vi "Gera_Dmd_Frame.vi"(8 "i":i32, 9 "c_Stop":bool, 11 "A2K - RT":dbl[](array[numeric])) -> (3 "a2c_serial":u8[](array[numeric]))   [LabVIEW 2011]
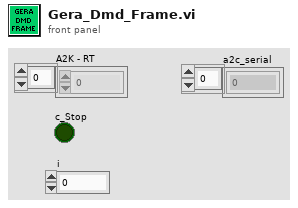
[diagram p1: front panel]
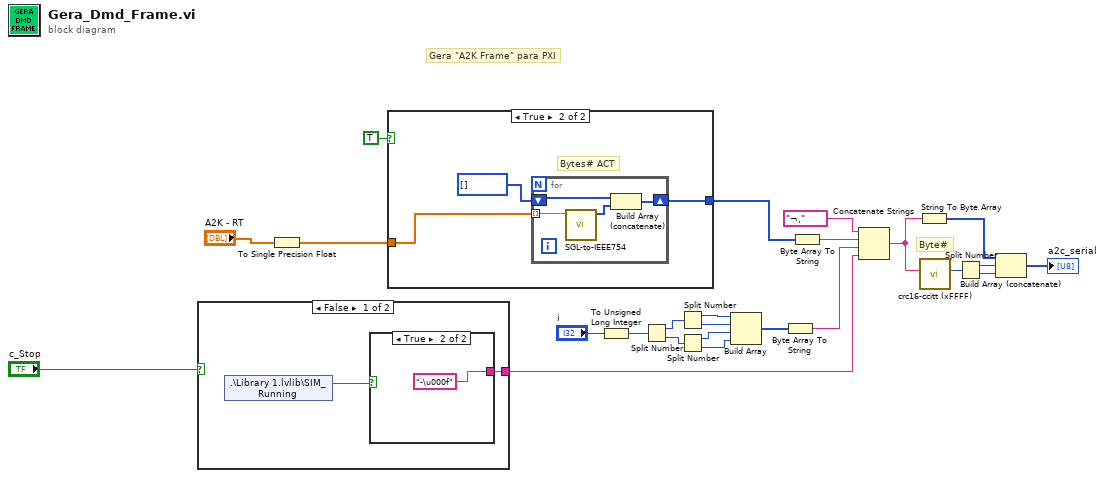
[diagram p0: block diagram]
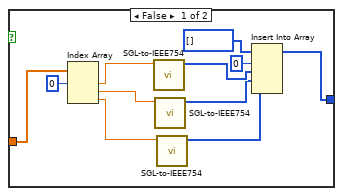
[diagram p2: hidden frame]
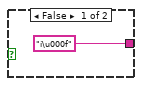
[diagram p3: hidden frame]
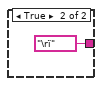
[diagram p4: hidden frame]
diagram:
  # "Byte#"
  # "Gera \"A2K Frame\" para PXI"
  n1 = case shown="False" "c_Stop" {
    tunnel: [w26 "\rï"] -> w18
    frame False {
      n2 = shared-variable ".\\Library 1.lvlib\\SIM_Running"() -> (w25:bool)  [unwired: 1 in, 1 out]
      n3 = case shown="True" w25 {
        tunnel: ["í\u000f" "­\u000f"] -> w26
        frame False {
        }
        frame True {
        }
      }
    }
    frame True {
    }
  }
  n4 = To Single Precision Float(number="A2K - RT") -> (single precision float=w19:sgl[])
  n5 = case shown="True" TRUE {
    tunnel: [w30 w43] -> w20
    tunnel: w19 -> [w40 w41]
    frame False {
      n6 = Index Array(array=w40, index #1=0 ("index")) -> (element #1=w39:sgl, element #2=w37:sgl, element #3=w36:sgl)  [unwired: 2 in]
      n7 = call "SGL-to-IEEE754.vi"("Input_DBL"=w39) -> ("Output_U8"=w33:u8[])  [unwired: 10 in]
      n8 = call "SGL-to-IEEE754.vi"("Input_DBL"=w37) -> ("Output_U8"=w32:u8[])  [unwired: 10 in]
      n9 = call "SGL-to-IEEE754.vi"("Input_DBL"=w36) -> ("Output_U8"=w31:u8[])  [unwired: 10 in]
      n10 = Insert Into Array(array=u8[] [] ("Output_U8"), index=0, new element #1=w33, new element #2=w32, new element #3=w31) -> (w30:u8[])
    }
    frame True {
      # "Bytes# ACT"
      n11 = for {
        tunnel: w41 -> [w47] mode=indexing
        shift-right: [w44] -> w43
        shift-left: u8[] [] ("Output_U8") -> [w45]
        n12 = call "SGL-to-IEEE754.vi"("Input_DBL"=w47) -> ("Output_U8"=w46:u8[])  [unwired: 10 in]
        n13 = Build Array (concatenate)(w45, w46) -> (w44:u8[])
      }
    }
  }
  n14 = To Unsigned Long Integer(number="i") -> (unsigned 32bit integer=w11:u32)
  n15 = Split Number(x=w11) -> (hi(x)=w9:u16, lo(x)=w10:u16)
  n16 = Split Number(x=w9) -> (hi(x)=w8:u8, lo(x)=w7:u8)
  n17 = Split Number(x=w10) -> (hi(x)=w6:u8, lo(x)=w5:u8)
  n18 = Build Array(w8, w7, w6, w5) -> (w4:u8[])
  n19 = Byte Array To String(unsigned byte array=w4) -> (string=w3:string)
  n20 = Byte Array To String(unsigned byte array=w20) -> (string=w12:string)
  n21 = Concatenate Strings("¬,", w12, w3, w18) -> (w24:string)
  n22 = String To Byte Array(string=w24) -> (unsigned byte array=w17:u8[])
  n23 = call "crc16-ccitt (xFFFF).vi"("Message"=w24) -> ("CRC"=w23:u16)  [unwired: 9 in, 1 out]
  n24 = Split Number(x=w23) -> (hi(x)=w22:u8, lo(x)=w21:u8)
  n25 = Build Array (concatenate)(w17, w22, w21) -> (→"a2c_serial":u8[])
